vi "Copy Test.vi"(4 "New ID":string, 6 "Move?":bool, 7 "New Parent ID":string, 8 "error in (no error)":errorcluster, 9 "Insertion Index":i32=-1, 10 "Test ID":string, 11 "Test Executive Ref":refnum<data-value>) -> (0 "error out":errorcluster, 2 "Test ID out":string, 3 "Test Executive Ref out":refnum<data-value>)   [LabVIEW 2020, in "Test Executive.lvlib" / "TestExecutive Ref.lvclass"]
uses:
  <vilib>/gpm_packages/@cs/test-executive/Source/Test Executive/TestExecutive Ref/TestExecutive Ref.lvclass
  <vilib>/gpm_packages/@cs/test-executive/Source/Test Executive/ITestExecutive/ITest Executive.lvclass
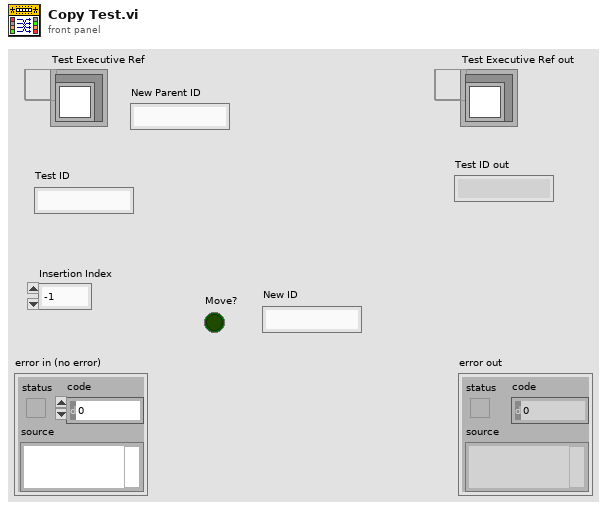
[diagram p1: front panel]
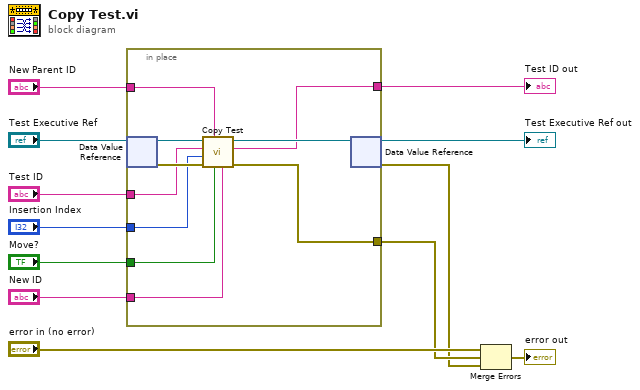
[diagram p0: block diagram]
diagram:
  n1 = in-place {
    in-place-border: "New Parent ID" -> [w20]
    in-place-border: [w19] -> w9
    in-place-border: "Test ID" -> [w17]
    in-place-border: "Insertion Index" -> [w16]
    in-place-border: "Move?" -> [w15]
    in-place-border: "New ID" -> [w14]
    in-place-border: [w13] -> w1
    n2 = in-place-dvr #1("Test Executive Ref") -> (w22:refnum<class "ITest Executive.lvclass">, w18:errorcluster)
    n3 = call-dynamic "Copy Test.vi"("New ID"=w14, "Move?"=w15, "New Parent ID"=w20, "error in (no error)"=w18, "Insertion Index"=w16, "Test ID"=w17, "ITest Executive in"=w22) -> ("error out"=w19:errorcluster, "Test ID out"=w13:string, "ITest Executive out"=w21:refnum<class "ITest Executive.lvclass">)  [unwired: 2 in]
    n4 = in-place-dvr #1(w21) -> (→"Test Executive Ref out":refnum<data-value>, w8:errorcluster)
  }
  "Test ID out" <- w1
  n5 = Merge Errors("error in (no error)", w9, w8) -> (→"error out":errorcluster)
